vi "Get Path for Scripts.vi"(8 "error in (no error)":errorcluster, 11 "Kasli in":refnum<class "Kasli.lvclass">) -> (0 "error out":errorcluster, 1 "File pattern":string="*.py", 2 "Path":path, 3 "Kasli out":refnum<class "Kasli.lvclass">)   [LabVIEW 2020, in "TALOS.lvlib" / "Kasli Wrapper 2.0.lvlib" / "Kasli.lvclass"]
uses:
  Kasli.lvclass
  Kasli.lvclass/Kasli.ctl
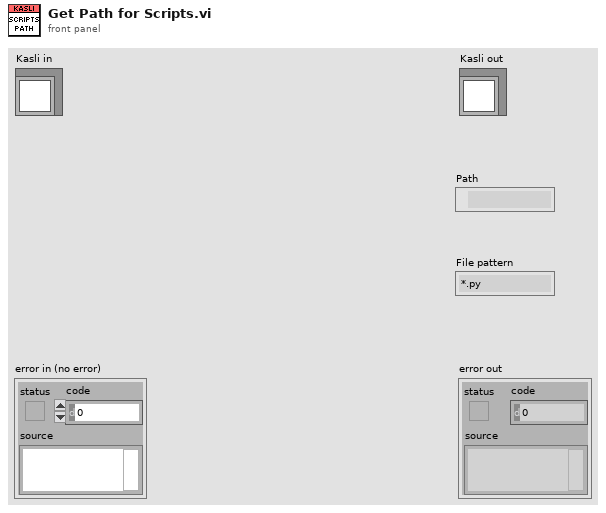
[diagram p1: front panel]
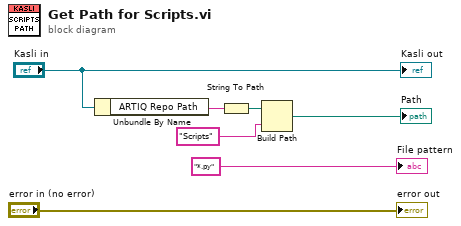
[diagram p0: block diagram]
diagram:
  n1 = Unbundle By Name("Kasli in") -> ("ARTIQ Repo Path"=w3:string)
  n2 = String To Path(string=w3) -> (path=w4:path)
  n3 = Build Path(base path=w4, name or relative path="Scripts" ("ARTIQ Repo Path")) -> (appended path=→"Path":path)
  "error out" <- "error in (no error)"
  "Kasli out" <- "Kasli in"
  "File pattern" <- "*.py" ("ARTIQ Repo Path")
